vi "AB_Engine_Make_App_Flags.vi"(8 "App Compatibility Mode":bool, 9 "enable debugging":bool, 10 "cmd line arg":bool, 11 "LabVIEW RT?":bool) -> (2 "AppFlags":u32 format="%.0x")   [LabVIEW 2020]
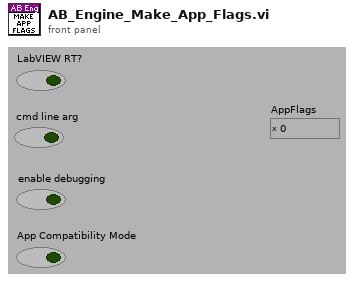
[diagram p1: front panel]
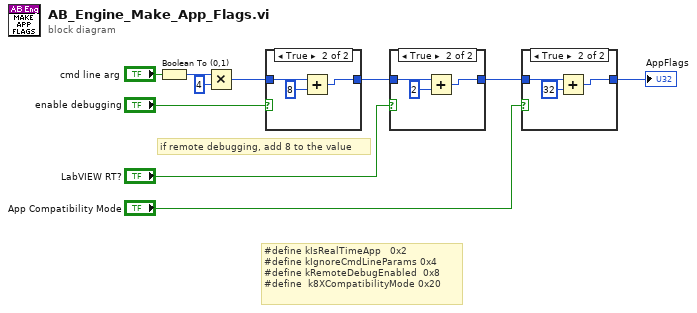
[diagram p0: block diagram]
diagram:
  # "#define kIsRealTimeApp\t\t\t0x2\n#define kIgnoreCmdLineParams\t0x4\n#define kRemoteDebugEnabled\t\t0x8\n#define  k8XCompatibilityMode 0x20"
  # "if remote debugging, add 8 to the value"
  n1 = Boolean To (0,1)(Boolean="cmd line arg") -> (0, 1=w10:i16)
  n2 = Multiply(x=w10, y=u32 4) -> (x*y=w7:u32)
  n3 = case shown="True" "enable debugging" {
    tunnel: w7 -> [w11 w13]
    tunnel: [w11 w12] -> w5
    frame False {
    }
    frame True {
      n4 = Add(x=w13, y=u32 8) -> (x+y=w12:u32)
    }
  }
  n5 = case shown="True" "LabVIEW RT?" {
    tunnel: w5 -> [w15 w17]
    tunnel: [w15 w16] -> w3
    frame False {
    }
    frame True {
      n6 = Add(x=w17, y=u32 2) -> (x+y=w16:u32)
    }
  }
  n7 = case shown="True" "App Compatibility Mode" {
    tunnel: w3 -> [w19 w21]
    tunnel: [w19 w20] -> w2
    frame False {
    }
    frame True {
      n8 = Add(x=w21, y=u32 32) -> (x+y=w20:u32)
    }
  }
  "AppFlags" <- w2
